vi "SpotFindResults.vi"(4 "Spots in":T1[](array[typedef]) {"F2-Value overall" format="%.2f"; "tauerror" format="%.2f"; "Lifetime[ns]" format="%.2f"; "F2-Value TAC" format="%.2f"}, 5 "set?":bool) -> (1 "Spots out":T1[](array[typedef]) {"F2-Value overall" format="%.2f"; "tauerror" format="%.2f"; "Lifetime[ns]" format="%.2f"; "F2-Value TAC" format="%.2f"})   [LabVIEW 2009]
uses:
  spotproperties.ctl
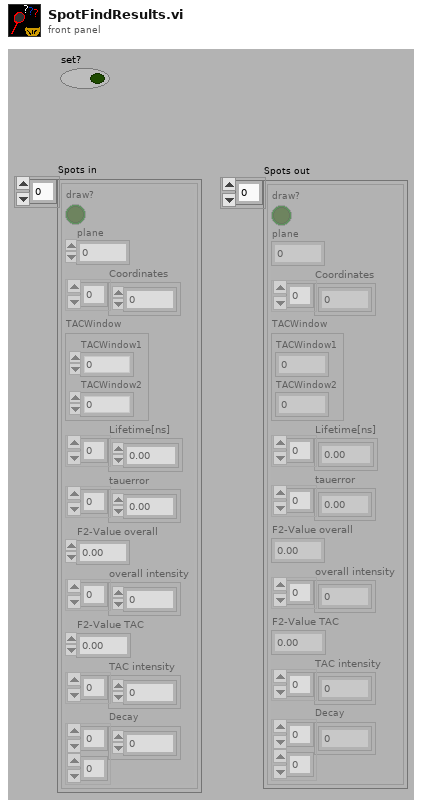
[diagram p1: front panel]
types:
  T1 = typedef "spotproperties.ctl" = cluster{"draw?":bool, "plane":u32, "Coordinates":i32[], "TACWindow":cluster{"TACWindow1":i32, "TACWindow2":i32}, "Lifetime[ns]":ext[], "tauerror":dbl[], "F2-Value overall":dbl, "overall intensity":u32[], "F2-Value TAC":dbl, "TAC intensity":u32[], "Decay":u32[][]}
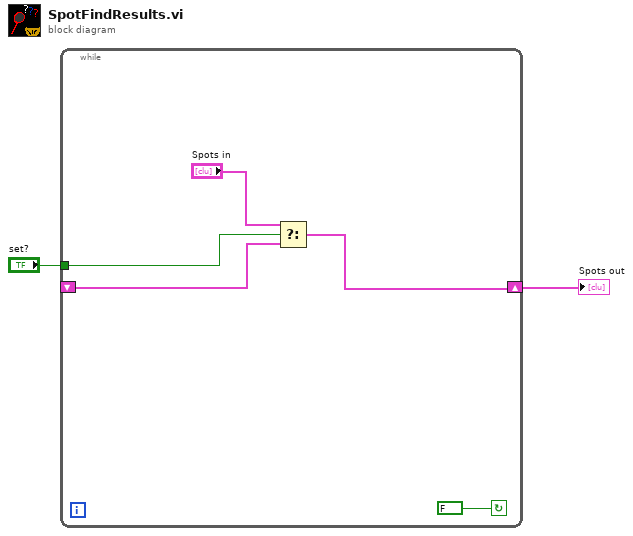
[diagram p0: block diagram]
diagram:
  n1 = while {
    tunnel: "set?" -> [w6]
    shift-right: [w3] -> w1
    shift-left: _ -> [w5]
    stop <- FALSE continue-if-true
    n2 = Select(t="Spots in", s=w6, f=w5) -> (s? t:f=w3:T1[])
  }
  "Spots out" <- w1
